vi "WRITE - Wave File.vi"(5 "error in (no error)":errorcluster, 6 "Scaling Factor":dbl=1.0, 7 "wForms":waveform(dbl)[](array[waveform]), 8 "Filename Option":T2(ring), 9 "Path":path, 10 "Multi Signal Save Option":T1, 11 "Filename":string, 12 "Fade IN and OUT":bool) -> (19 "error out":errorcluster)   [LabVIEW 2022 SP3, in "WaveFile.lvclass"]
uses:
  WaveFile.lvclass
  protected/Multi Signals Save Option.ctl
  <vilib>/sound2/lvsound2.llb/Sound Data Format.ctl
  <vilib>/sound2/lvsound2.llb/Sound File Write Open.vi
  <vilib>/sound2/lvsound2.llb/Sound File Write (DBL Single).vi
  <vilib>/sound2/lvsound2.llb/Sound File Write (DBL).vi
  API/GSwFormDSP_class/GSwFormDSP.lvclass
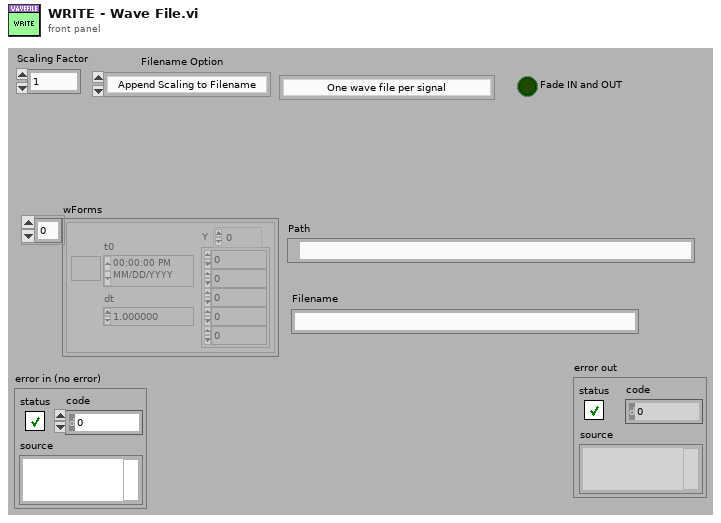
[diagram p1: front panel]
types:
  T1 = typedef "WaveFile.lvclass/Multi Signals Save Option.ctl" = enum16{"One wave file per signal", "Concatenate ALL signals to a single file", "Stereo (Ch1 is Left, Ch2 is Right)", "Stereo (Ch1 is Right, Ch2 is Left)"}
  T2 = enum16{"Append Scaling to Filename", "No Scaling Info"}
  T3 = enum16{"Fade IN and OUT", "Fade IN ONLY", "Fade OUT ONLY", "None"}
  T4 = typedef "Sound Data Format.ctl" = cluster{"sample rate (S/s)":dbl, "number of channels":i32, "bits per sample":i32}
  T5 = typedef "Sound File Refnum.ctl" = refnum<file>
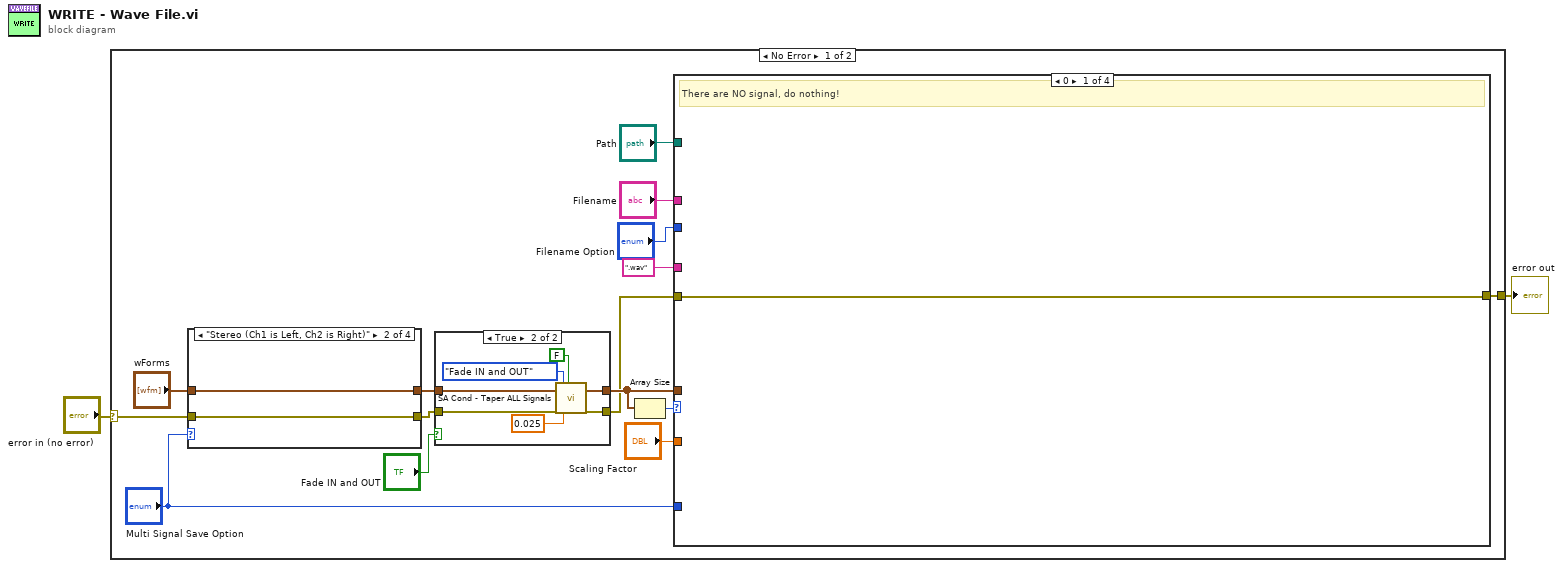
[diagram p0: block diagram]
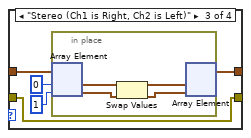
[diagram p4: hidden frame]
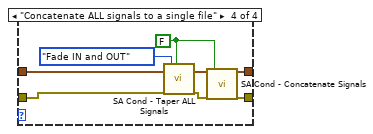
[diagram p5: hidden frame]
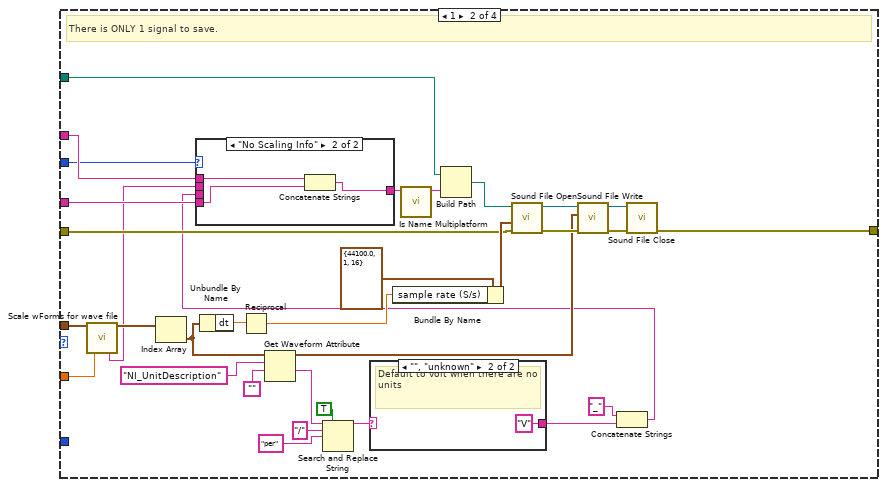
[diagram p6: hidden frame]
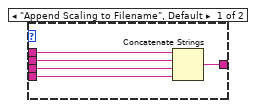
[diagram p7: hidden frame]
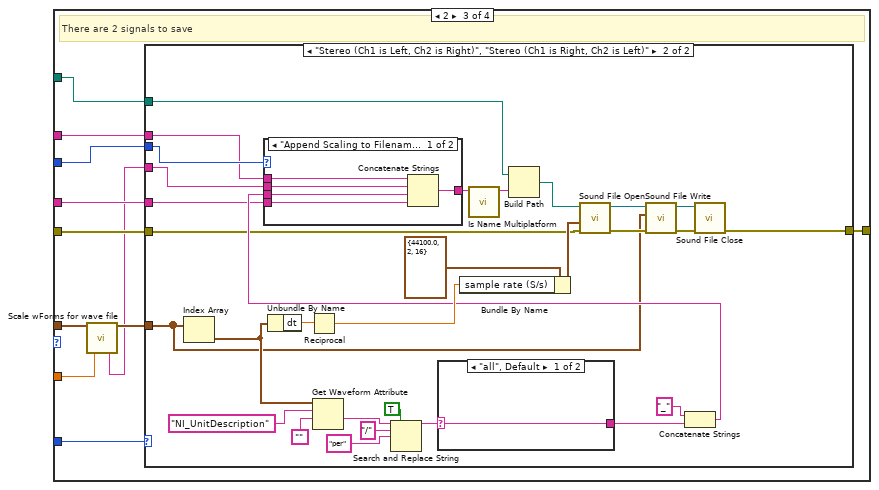
[diagram p9: hidden frame]
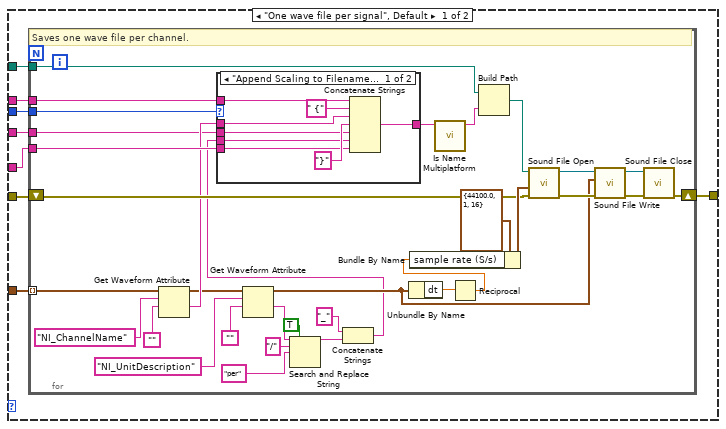
[diagram p10: hidden frame]
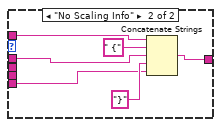
[diagram p11: hidden frame]
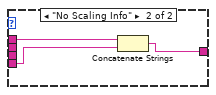
[diagram p12: hidden frame]
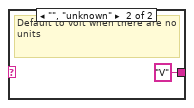
[diagram p13: hidden frame]
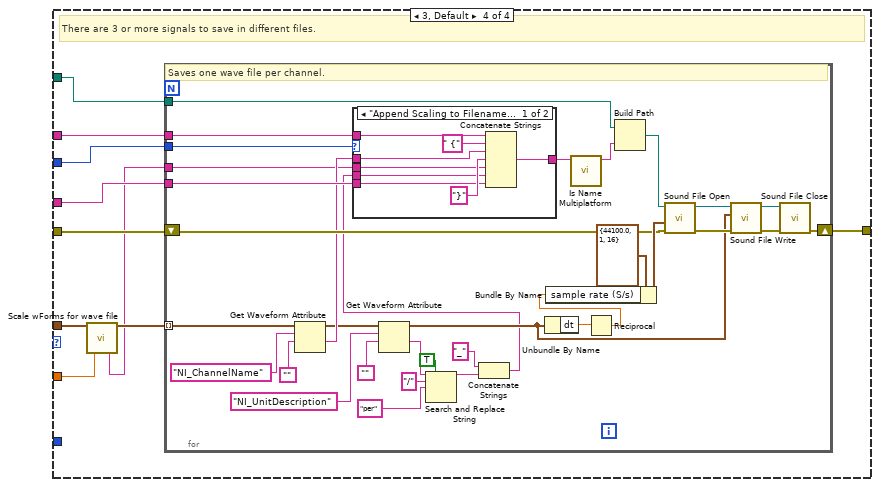
[diagram p14: hidden frame]
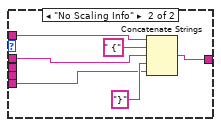
[diagram p15: hidden frame]
diagram:
  n1 = case shown="No Error" "error in (no error)" {
    selector: "error in (no error)" -> [w9 w255]
    tunnel: [w15 w255] -> w1
    frame No Error {
      n2 = case shown="\"Stereo (Ch1 is Left, Ch2 is Right)\"" "Multi Signal Save Option" {
        tunnel: [w28 w29 w31 w43] -> w8
        tunnel: "wForms" -> [w28 w29 w35 w44]
        tunnel: w9 -> [w27 w30 w34 w42]
        tunnel: [w27 w30 w34 w40] -> w6
        frame "One wave file per signal", Default {
        }
        frame "Stereo (Ch1 is Left, Ch2 is Right)" {
        }
        frame "Stereo (Ch1 is Right, Ch2 is Left)" {
          n3 = in-place {
            n4 = in-place-array #1(w35, 0, 1) -> (w39:waveform(dbl), w37:waveform(dbl))
            n5 = Swap Values(12:w39, 14:w37) -> (1:w38:waveform(dbl), 3:w36:waveform(dbl))  [unwired: 1 in]
            n6 = in-place-array #1(w38, w36) -> (w31:waveform(dbl)[])  [unwired: 2 out]
          }
        }
        frame "Concatenate ALL signals to a single file" {
          w47 = FALSE ("Anotate Signal Name")
          n7 = call "SA Cond - Taper ALL Signals.vi"("wForm IN"=w44, "error in (no error)"=w42, "Fade Options"=T3."Fade IN and OUT", "Anotate Signal Name"=w47) -> ("wForm OUT"=w46:waveform(dbl)[], "error out"=w41:errorcluster)  [unwired: 14 in]
          n8 = call "SA Cond - Concatenate Signals.vi"("Signal IN"=w46, "error in (no error)"=w41, "Anotate Signal Name"=w47) -> ("Signal OUT"=w43:waveform(dbl)[], "error out"=w40:errorcluster)  [unwired: 15 in]
        }
      }
      n9 = case shown="True" "Fade IN and OUT" {
        tunnel: [w19 w24] -> w7
        tunnel: w8 -> [w19 w26]
        tunnel: w6 -> [w18 w22]
        tunnel: [w18 w21] -> w5
        frame False {
        }
        frame True {
          n10 = call "SA Cond - Taper ALL Signals.vi"("wForm IN"=w26, "error in (no error)"=w22, "Fade Options"=T3."Fade IN and OUT", "Time for Fade IN/OUT (sec)"=0.025, "Anotate Signal Name"=FALSE) -> ("wForm OUT"=w24:waveform(dbl)[], "error out"=w21:errorcluster)  [unwired: 13 in]
        }
      }
      n11 = Array Size(array=w7) -> (size(s)=w16:i32)
      n12 = case shown="0" w16 {
        tunnel: "Path" -> [_ w71 w100 w205]
        tunnel: w7 -> [_ w65 w97 w202]
        tunnel: w5 -> [w48 w73 w102 w207]
        tunnel: [w48 w72 w101 w206] -> w15
        tunnel: "Filename" -> [_ w69 w99 w204]
        tunnel: ".wav" ("string") -> [_ w68 w98 w203]
        tunnel: "Scaling Factor" -> [_ w63 w95 w200]
        tunnel: "Filename Option" -> [_ w49 w93 w198]
        tunnel: "Multi Signal Save Option" -> [_ _ w92 _]
        frame 0 {
          # "There are NO signal, do nothing!"
        }
        frame 1 {
          # "There is ONLY 1 signal to save."
          n13 = call "Scale wForms for wave file.vi"("Signal IN"=w65, "Desired Level (EU)"=w63) -> ("Ref Label"=w53:string, "Signal OUT"=w64:waveform(dbl)[])  [unwired: 16 in]
          n14 = Index Array(array=w64) -> (element=w55:waveform(dbl))  [unwired: 1 in]
          n15 = Unbundle By Name(w55) -> ("dt"=w75:dbl)
          n16 = Reciprocal(x=w75) -> (1/x=w74:dbl)
          n17 = Get Waveform Attribute(5:"", 6:"NI_UnitDescription" ("Att - wform unit"), 7:w55) -> (1:w59:string, 3:w54:waveform(dbl))  [unwired: 1 in, 2 out]
          n18 = Search and Replace String(replace all?=TRUE ("replace all? (F)"), input string=w59, search string="/", replace string="per" ("replace string (\"\")")) -> (result string=w51:string)  [unwired: 4 in, 3 out]
          n19 = case shown="\"\", \"unknown\"" w51 {
            selector: w51 -> [w90 _]
            tunnel: [w90 "V"] -> w50
            frame "all", Default {
            }
            frame "", "unknown" {
              # "Default to volt when there are no units"
            }
          }
          n20 = Bundle By Name(cluster=T4 {"sample rate (S/s)"=44100.0, "number of channels"=1, "bits per sample"=16} ("sound format"), "sample rate (S/s)"=w74) -> (w76:T4)
          n21 = Concatenate Strings("_" ("search string"), w50) -> (w52:string)
          n22 = case shown="\"No Scaling Info\"" w49 {
            tunnel: w69 -> [w86 w89]
            tunnel: w68 -> [w85 w88]
            tunnel: [w84 w87] -> w67
            tunnel: w53 -> [w83 _]
            tunnel: w52 -> [w82 _]
            frame "Append Scaling to Filename", Default {
              n23 = Concatenate Strings(w86, w83, w82, w85) -> (w84:string)
            }
            frame "No Scaling Info" {
              n24 = Concatenate Strings(w89, w88) -> (w87:string)
            }
          }
          n25 = call <vilib>:"Is Name Multiplatform.vi"("filename"=w67) -> ("suggested filename"=w66:string)  [unwired: 6 in, 4 out]
          n26 = Build Path(base path=w71, name or relative path=w66) -> (appended path=w70:path)
          n27 = call-poly <vilib>:"Sound File Open.vi"("error in (no error)"=w73, "sound format"=w76, "path"=w70) -> ("error out"=w81:errorcluster, "sound file refnum"=w80:T5)  [unwired: 7 in]
          n28 = call-poly <vilib>:"Sound File Write.vi"("error in (no error)"=w81, "data"=w54, "sound file refnum"=w80) -> ("error out"=w79:errorcluster, "sound file refnum out"=w78:T5)  [unwired: 7 in]
          n29 = call <vilib>:"Sound File Close.vi"("error in (no error)"=w79, "sound file refnum"=w78) -> ("error out"=w72:errorcluster)  [unwired: 9 in]
        }
        frame 2 {
          # "There are 2 signals to save"
          n30 = call "Scale wForms for wave file.vi"("Signal IN"=w97, "Desired Level (EU)"=w95) -> ("Ref Label"=w94:string, "Signal OUT"=w96:waveform(dbl)[])  [unwired: 16 in]
          n31 = case shown="\"Stereo (Ch1 is Left, Ch2 is Right)\", \"Stereo (Ch1 is Right, Ch2 is Left)\"" w92 {
            tunnel: w102 -> [w110 w162]
            tunnel: [w109 w163] -> w101
            tunnel: w100 -> [w108 w164]
            tunnel: w99 -> [w107 w159]
            tunnel: w98 -> [w106 w161]
            tunnel: w96 -> [w105 w158]
            tunnel: w94 -> [w104 w160]
            tunnel: w93 -> [w103 w165]
            frame "One wave file per signal", Default {
              n32 = for {
                tunnel: w105 -> [w129] mode=indexing
                shift-right: [w134] -> w109
                shift-left: w110 -> [w135]
                tunnel: w108 -> [w133]
                tunnel: w107 -> [w131]
                tunnel: w106 -> [w130]
                tunnel: w104 -> [w123]
                tunnel: w103 -> [w111]
                # "Saves one wave file per channel."
                n33 = Get Waveform Attribute(5:"", 6:"NI_ChannelName" ("Att - wform Name"), 7:w129) -> (1:w126:string, 3:w121:waveform(dbl))  [unwired: 1 in, 2 out]
                n34 = Get Waveform Attribute(5:"", 6:"NI_UnitDescription" ("Att - wform unit"), 7:w121) -> (1:w117:string, 3:w120:waveform(dbl))  [unwired: 1 in, 2 out]
                n35 = Search and Replace String(replace all?=TRUE ("replace all? (F)"), input string=w117, search string="/", replace string="per" ("replace string (\"\")")) -> (result string=w113:string)  [unwired: 4 in, 3 out]
                n36 = Concatenate Strings("_" ("search string"), w113) -> (w112:string)
                n37 = case shown="\"Append Scaling to Filename\", Default" w111 {
                  tunnel: w131 -> [w151 w155]
                  tunnel: w130 -> [w148 w153]
                  tunnel: w126 -> [w147 w154]
                  tunnel: [w146 w152] -> w125
                  tunnel: w123 -> [w145 _]
                  tunnel: w112 -> [w144 _]
                  frame "Append Scaling to Filename", Default {
                    n38 = Concatenate Strings(w151, " {" ("string"), w147, "}" ("string"), w145, w144, w148) -> (w146:string)
                  }
                  frame "No Scaling Info" {
                    n39 = Concatenate Strings(w155, " {" ("string"), w154, "}" ("string"), w153) -> (w152:string)
                  }
                }
                n40 = Unbundle By Name(w120) -> ("dt"=w137:dbl)
                n41 = call <vilib>:"Is Name Multiplatform.vi"("filename"=w125) -> ("suggested filename"=w124:string)  [unwired: 6 in, 4 out]
                n42 = Reciprocal(x=w137) -> (1/x=w136:dbl)
                n43 = Bundle By Name(cluster=T4 {"sample rate (S/s)"=44100.0, "number of channels"=1, "bits per sample"=16} ("sound format"), "sample rate (S/s)"=w136) -> (w138:T4)
                n44 = Build Path(base path=w133, name or relative path=w124) -> (appended path=w132:path)
                n45 = call-poly <vilib>:"Sound File Open.vi"("error in (no error)"=w135, "sound format"=w138, "path"=w132) -> ("error out"=w143:errorcluster, "sound file refnum"=w142:T5)  [unwired: 7 in]
                n46 = call-poly <vilib>:"Sound File Write.vi"("error in (no error)"=w143, "data"=w120, "sound file refnum"=w142) -> ("error out"=w141:errorcluster, "sound file refnum out"=w140:T5)  [unwired: 7 in]
                n47 = call <vilib>:"Sound File Close.vi"("error in (no error)"=w141, "sound file refnum"=w140) -> ("error out"=w134:errorcluster)  [unwired: 9 in]
              }
            }
            frame "Stereo (Ch1 is Left, Ch2 is Right)", "Stereo (Ch1 is Right, Ch2 is Left)" {
              n48 = Index Array(array=w158) -> (element=w169:waveform(dbl))  [unwired: 1 in]
              n49 = Unbundle By Name(w169) -> ("dt"=w181:dbl)
              n50 = Reciprocal(x=w181) -> (1/x=w180:dbl)
              n51 = Get Waveform Attribute(5:"", 6:"NI_UnitDescription" ("Att - wform unit"), 7:w169) -> (1:w173:string)  [unwired: 1 in, 3 out]
              n52 = Search and Replace String(replace all?=TRUE ("replace all? (F)"), input string=w173, search string="/", replace string="per" ("replace string (\"\")")) -> (result string=w167:string)  [unwired: 4 in, 3 out]
              n53 = case shown="\"all\", Default" w167 {
                selector: w167 -> [w196 _]
                tunnel: [w196 "V"] -> w166
                frame "all", Default {
                }
                frame "", "unknown" {
                  # "Default to volt when there are no units"
                }
              }
              n54 = Bundle By Name(cluster=T4 {"sample rate (S/s)"=44100.0, "number of channels"=2, "bits per sample"=16} ("sound format"), "sample rate (S/s)"=w180) -> (w182:T4)
              n55 = Concatenate Strings("_" ("search string"), w166) -> (w168:string)
              n56 = case shown="\"Append Scaling to Filename\", Default" w165 {
                tunnel: w159 -> [w192 w195]
                tunnel: w161 -> [w191 w194]
                tunnel: [w190 w193] -> w178
                tunnel: w160 -> [w189 _]
                tunnel: w168 -> [w188 _]
                frame "Append Scaling to Filename", Default {
                  n57 = Concatenate Strings(w192, w189, w188, w191) -> (w190:string)
                }
                frame "No Scaling Info" {
                  n58 = Concatenate Strings(w195, w194) -> (w193:string)
                }
              }
              n59 = call <vilib>:"Is Name Multiplatform.vi"("filename"=w178) -> ("suggested filename"=w177:string)  [unwired: 6 in, 4 out]
              n60 = Build Path(base path=w164, name or relative path=w177) -> (appended path=w179:path)
              n61 = call-poly <vilib>:"Sound File Open.vi"("error in (no error)"=w162, "sound format"=w182, "path"=w179) -> ("error out"=w187:errorcluster, "sound file refnum"=w186:T5)  [unwired: 7 in]
              n62 = call-poly <vilib>:"Sound File Write.vi"("error in (no error)"=w187, "data"=w158, "sound file refnum"=w186) -> ("error out"=w185:errorcluster, "sound file refnum out"=w184:T5)  [unwired: 7 in]
              n63 = call <vilib>:"Sound File Close.vi"("error in (no error)"=w185, "sound file refnum"=w184) -> ("error out"=w163:errorcluster)  [unwired: 9 in]
            }
          }
        }
        frame 3, Default {
          # "There are 3 or more signals to save in different files."
          n64 = call "Scale wForms for wave file.vi"("Signal IN"=w202, "Desired Level (EU)"=w200) -> ("Ref Label"=w199:string, "Signal OUT"=w201:waveform(dbl)[])  [unwired: 16 in]
          n65 = for {
            tunnel: w201 -> [w226] mode=indexing
            shift-right: [w231] -> w206
            shift-left: w207 -> [w232]
            tunnel: w205 -> [w230]
            tunnel: w204 -> [w228]
            tunnel: w203 -> [w227]
            tunnel: w199 -> [w220]
            tunnel: w198 -> [w208]
            # "Saves one wave file per channel."
            n66 = Get Waveform Attribute(5:"", 6:"NI_ChannelName" ("Att - wform Name"), 7:w226) -> (1:w223:string, 3:w218:waveform(dbl))  [unwired: 1 in, 2 out]
            n67 = Get Waveform Attribute(5:"", 6:"NI_UnitDescription" ("Att - wform unit"), 7:w218) -> (1:w214:string, 3:w217:waveform(dbl))  [unwired: 1 in, 2 out]
            n68 = Search and Replace String(replace all?=TRUE ("replace all? (F)"), input string=w214, search string="/", replace string="per" ("replace string (\"\")")) -> (result string=w210:string)  [unwired: 4 in, 3 out]
            n69 = Concatenate Strings("_" ("search string"), w210) -> (w209:string)
            n70 = case shown="\"Append Scaling to Filename\", Default" w208 {
              tunnel: w228 -> [w248 w252]
              tunnel: w227 -> [w245 w250]
              tunnel: w223 -> [w244 w251]
              tunnel: [w243 w249] -> w222
              tunnel: w220 -> [w242 _]
              tunnel: w209 -> [w241 _]
              frame "Append Scaling to Filename", Default {
                n71 = Concatenate Strings(w248, " {" ("string"), w244, "}" ("string"), w242, w241, w245) -> (w243:string)
              }
              frame "No Scaling Info" {
                n72 = Concatenate Strings(w252, " {" ("string"), w251, "}" ("string"), w250) -> (w249:string)
              }
            }
            n73 = Unbundle By Name(w217) -> ("dt"=w234:dbl)
            n74 = call <vilib>:"Is Name Multiplatform.vi"("filename"=w222) -> ("suggested filename"=w221:string)  [unwired: 6 in, 4 out]
            n75 = Reciprocal(x=w234) -> (1/x=w233:dbl)
            n76 = Bundle By Name(cluster=T4 {"sample rate (S/s)"=44100.0, "number of channels"=1, "bits per sample"=16} ("sound format"), "sample rate (S/s)"=w233) -> (w235:T4)
            n77 = Build Path(base path=w230, name or relative path=w221) -> (appended path=w229:path)
            n78 = call-poly <vilib>:"Sound File Open.vi"("error in (no error)"=w232, "sound format"=w235, "path"=w229) -> ("error out"=w240:errorcluster, "sound file refnum"=w239:T5)  [unwired: 7 in]
            n79 = call-poly <vilib>:"Sound File Write.vi"("error in (no error)"=w240, "data"=w217, "sound file refnum"=w239) -> ("error out"=w238:errorcluster, "sound file refnum out"=w237:T5)  [unwired: 7 in]
            n80 = call <vilib>:"Sound File Close.vi"("error in (no error)"=w238, "sound file refnum"=w237) -> ("error out"=w231:errorcluster)  [unwired: 9 in]
          }
        }
      }
    }
    frame Error {
    }
  }
  "error out" <- w1
